vi "Run Main.vi"(8 "error in":errorcluster) -> (0 "error out":errorcluster)   [LabVIEW 2020, in "Hardware.lvlib"]
uses:
  Hardware.lvlib
  SubVIs and TypeDefs/Runtime Data.ctl
  Shared Ressources/gamepad-direction-enum.ctl
  Shared Ressources/Controller-button-pressed-enum.ctl
  <vilib>/Utility/inputDevices.llb/joystickAcquire.vi
  <userlib>/_OpenG.lib/array/array.llb/Search 1D Array (Boolean)__ogtk.vi
  <vilib>/Utility/inputDevices.llb/closeJoystick.vi
  Manager/Manager.lvlib
panel:
  out "Message Iterations":i32
  # "Message Handler: Run Main VI"
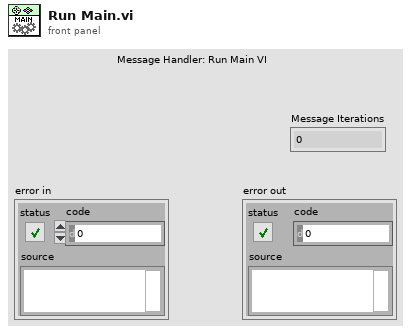
[diagram p1: front panel]
types:
  T1 = typedef "Hardware.lvlib/Runtime Data.ctl" = cluster{"ID":string, "connected?":bool, "System no.":i32, "device ID":refnum<k1>, "controller infos":cluster{"axes total":u32, "buttons total":u32, "pov total":u32, "device name":string}}
  T2 = typedef "Controller-button-pressed-enum.ctl" = enum16{"button 1", "button 2", "button 3", "button 4", "button 5", "button 6", "button 7", "button 8", "button 9", "button 10", "button 11", "button 12", "button 13", "button 14"}
  T3 = typedef "gamepad-direction-enum.ctl" = enum16{"Up Arrow", "Right Arrow", "Down Arrow", "Left Arrow"}
  T4 = cluster{"axes total":u32, "buttons total":u32, "pov total":u32, "device name":string}[]
  T5 = cluster{"axes total":u32, "buttons total":u32, "pov total":u32, "device name":string}
  T6 = cluster{"button 1":bool, "button 2":bool, "button 3":bool, "button 4":bool, "button 5":bool, "button 6":bool, "button 7":bool, "button 8":bool, "button 9":bool, "button 10":bool, "button 11":bool, "button 12":bool, "button 13":bool, "button 14":bool, "button 15":bool, "button 16":bool, "button 17":bool, "button 18":bool, "button 19":bool, "button 20":bool, "button 21":bool, "button 22":bool, "button 23":bool, "button 24":bool, "button 25":bool, "button 26":bool, "button 27":bool, "button 28":bool, "button 29":bool, "button 30":bool, "button 31":bool, "button 32":bool}
  T7 = cluster{"pov 1":i32, "pov 2":i32, "pov 3":i32, "pov 4":i32}
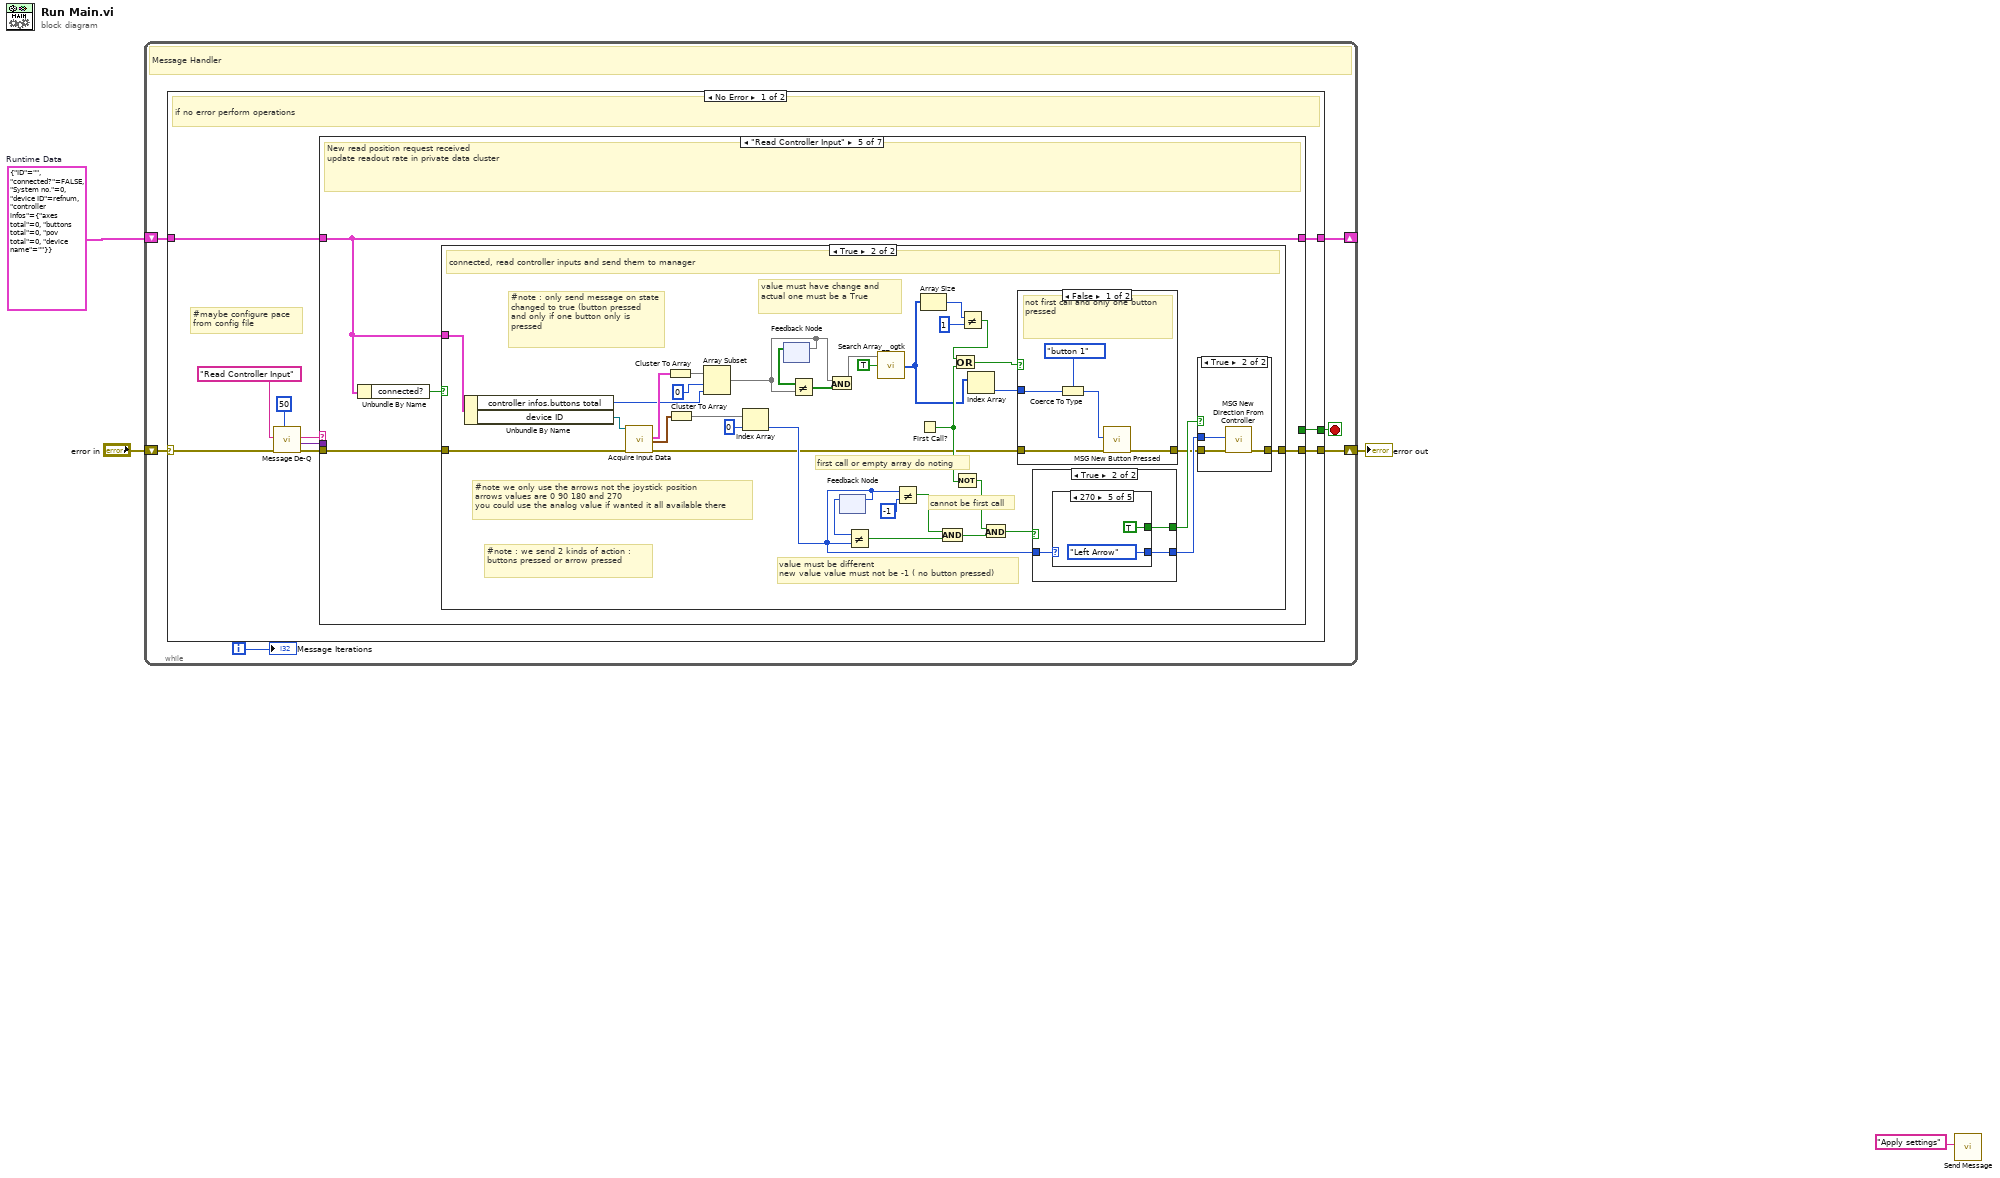
[diagram p0: block diagram]
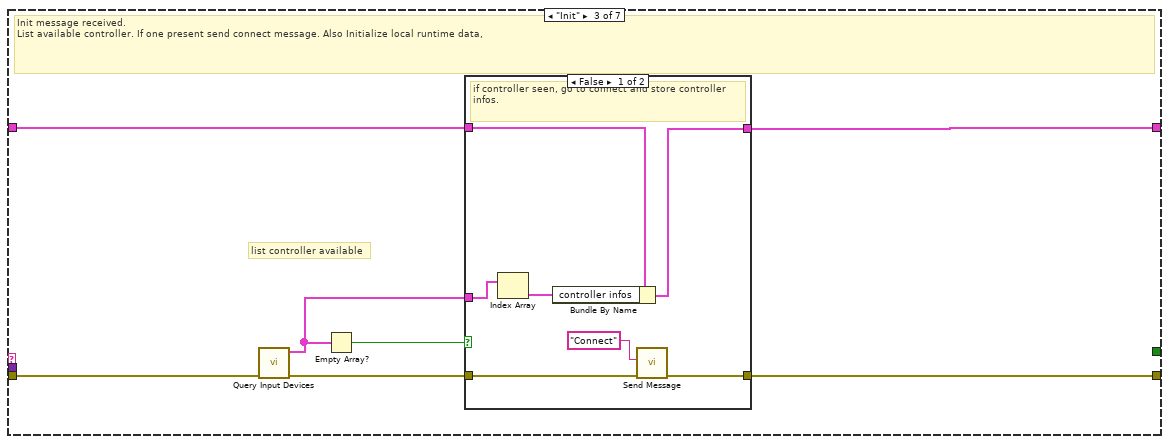
[diagram p4: hidden frame]
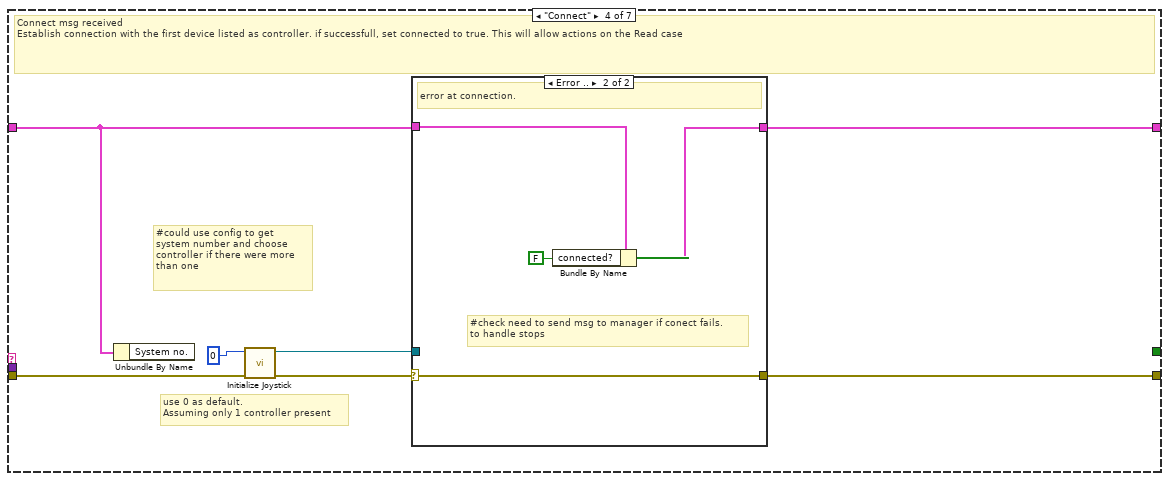
[diagram p6: hidden frame]
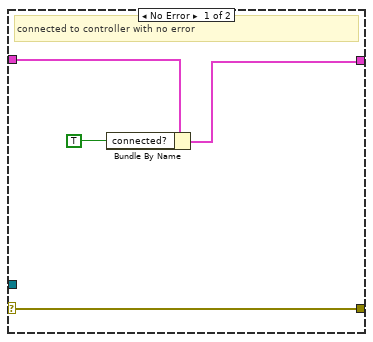
[diagram p7: hidden frame]
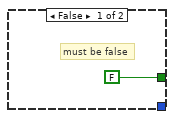
[diagram p11: hidden frame]
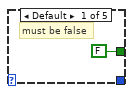
[diagram p12: hidden frame]
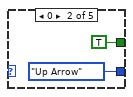
[diagram p13: hidden frame]
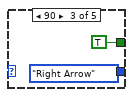
[diagram p14: hidden frame]
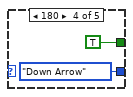
[diagram p15: hidden frame]
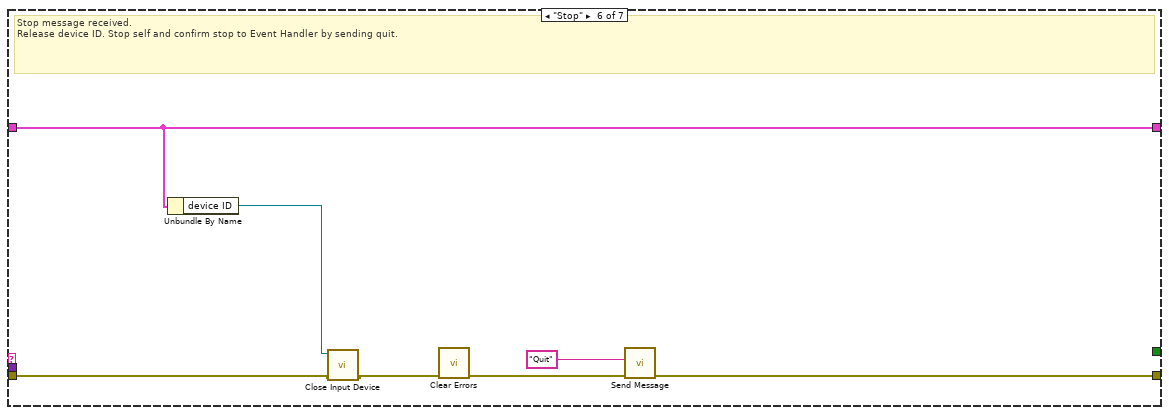
[diagram p16: hidden frame]
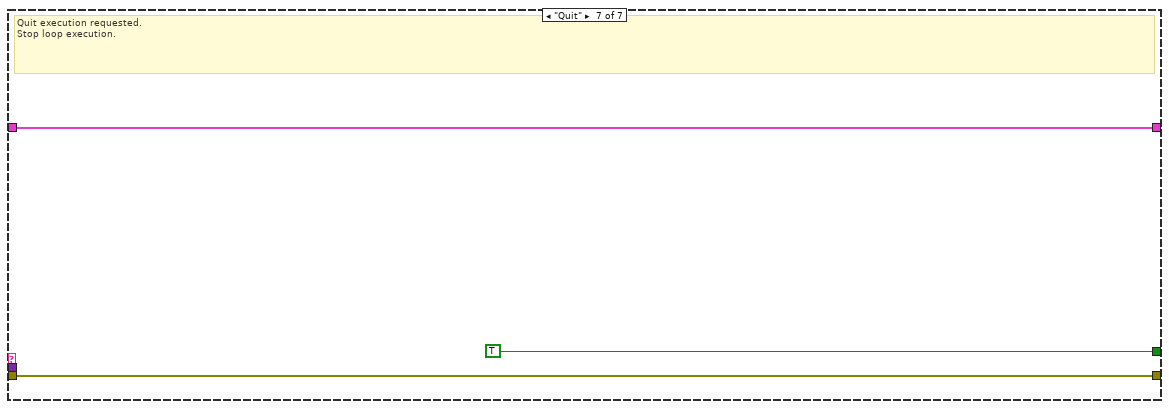
[diagram p17: hidden frame]
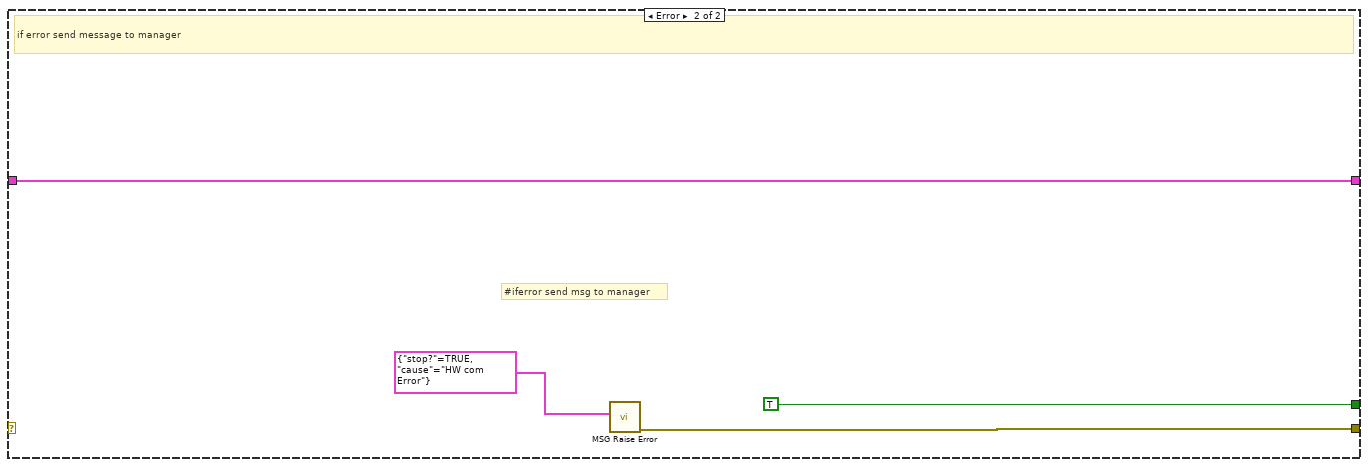
[diagram p18: hidden frame]
diagram:
  w1 = T1 {"ID"="", "connected?"=FALSE, "System no."=0, "device ID"=refnum, "controller infos"={"axes total"=0, "buttons total"=0, "pov total"=0, "device name"=""}}  # Runtime Data
  n1 = while {
    shift-right: [w8] -> w3
    shift-left: "error in" -> [w5]
    shift-right: [w6] -> _
    shift-left: w1 -> [w9]
    i -> [w10]
    stop <- w7 stop-if-true
    # "Message Handler"
    n2 = case shown="No Error" w5 {
      selector: w5 -> [w12 _]
      tunnel: w9 -> [w13 w131]
      tunnel: [w17 w129] -> w8
      tunnel: [w16 TRUE] -> w7
      tunnel: [w15 w131] -> w6
      frame No Error {
        # "#maybe configure pace\nfrom config file"
        # "if no error perform operations"
        n3 = call "Message De-Q.vi"("timeout [ms]"=50, "error in"=w12, "timeout cmd"="Read Controller Input") -> ("error out"=w18:errorcluster, "Payload"=w19:variant, "Command"=w20:string)  [unwired: 5 in, 1 out]
        n4 = case shown="\"Read Controller Input\"" w20 {
          tunnel: [w22 w23 w31 w47 w58 w124 w128] -> w17
          tunnel: w18 -> [w22 w23 w30 w44 w59 w120 w128]
          tunnel: [_ _ _ _ _ _ TRUE] -> w16
          tunnel: [w21 w24 w25 w46 w56 w123 w126] -> w15
          tunnel: w13 -> [w21 w24 w26 w41 w56 w123 w126]
          tunnel: w19 -> [_ _ _ _ _ _ _]
          frame Default {
            # "Message not recognized.\nDevelopment time error. Message not recognized. Maybe a typo? Pop up a blocking dialog for the developer to be informed about the situation."
          }
          frame "Message Timeout" {
            # "Message queue timeout.\nThis case is executed regularly when the messaging queue is empty.\nThink: IDLE."
          }
          frame "Init" {
            # "list controller available"
            # "Init message received.\nList available controller. If one present send connect message. Also Initialize local runtime data,"
            n5 = call <vilib>:"Query Input Devices.vi"("error in (no error)"=w30) -> ("error out"=w29:errorcluster, "joystick info"=w27:T4)  [unwired: 7 in, 2 out]
            n6 = Empty Array?(array=w27) -> (empty?=w28:bool)
            n7 = case shown="False" w28 {
              tunnel: [w37 w40] -> w31
              tunnel: w29 -> [w36 w40]
              tunnel: w27 -> [w35 _]
              tunnel: w26 -> [w33 w39]
              tunnel: [w32 w39] -> w25
              frame False {
                # "if controller seen, go to connect and store controller infos."
                n8 = Index Array(array=w35) -> (element=w34:T5)  [unwired: 1 in]
                n9 = Bundle By Name(cluster=w33, "controller infos"=w34) -> (w32:T1)
                n10 = call "Send Message.vi"("error in"=w36, "Command"="Connect") -> ("error out"=w37:errorcluster)  [unwired: 9 in]
              }
              frame True {
                # "#report no Controller connected"
              }
            }
          }
          frame "Connect" {
            # "use 0 as default.\nAssuming only 1 controller present"
            # "#could use config to get system number and choose controller if there were more than one"
            # "Connect msg received\nEstablish connection with the first device listed as controller. if successfull, set connected to true. This will allow actions on the Read case"
            n11 = Unbundle By Name(w41) -> ()  [unwired: 1 out]
            n12 = call <vilib>:"Initialize Joystick.vi"("error in (no error)"=w44, "device index"=0) -> ("error out"=w43:errorcluster, "device ID"=w42:refnum<k1>)  [unwired: 8 in]
            n13 = case shown="Error .." w43 {
              selector: w43 -> [w48 w55]
              tunnel: [w48 w55] -> w47
              tunnel: w41 -> [w51 w54]
              tunnel: [w50 w52] -> w46
              tunnel: w42 -> [_ _]
              frame No Error {
                # "connected to controller with no error"
                n14 = Bundle By Name(cluster=w51, "connected?"=TRUE) -> (w50:T1)
              }
              frame Error {
                # "#check need to send msg to manager if conect fails.\nto handle stops"
                # "error at connection."
                n15 = Bundle By Name(cluster=w54, "connected?"=FALSE) -> (w52:T1)
              }
            }
          }
          frame "Read Controller Input" {
            # "New read position request received\nupdate readout rate in private data cluster"
            n16 = Unbundle By Name(w56) -> ("connected?"=w57:bool)
            n17 = case shown="True" w57 {
              tunnel: w59 -> [w60 w95]
              tunnel: [w60 w72] -> w58
              tunnel: w56 -> [_ w94]
              frame False {
                # "not connected yet, do nothing"
              }
              frame True {
                # "#note : we send 2 kinds of action : buttons pressed or arrow pressed"
                # "#note we only use the arrows not the joystick position\narrows values are 0 90 180 and 270\nyou could use the analog value if wanted it all available there"
                # "#note : only send message on state changed to true (button pressed and only if one button only is pressed"
                # "cannot be first call"
                # "value must be different\nnew value value must not be -1 ( no button pressed)"
                # "first call or empty array do noting"
                # "value must have change and actual one must be a True"
                # "connected, read controller inputs and send them to manager"
                n18 = Unbundle By Name(w94) -> ("controller infos.buttons total"=w89:u32, "device ID"=w93:refnum<k1>)
                n19 = call-poly <vilib>:"Acquire Input Data.vi"("device ID"=w93, "error in (no error)"=w95) -> ("button info"=w92:T6, "direction info"=w88:T7, "error out"=w64:errorcluster)  [unwired: 13 in, 2 out]
                n20 = Cluster To Array(cluster=w92) -> (array=w91:bool[])
                n21 = Cluster To Array(cluster=w88) -> (array=w82:i32[])
                n22 = Array Subset(array=w91, index=0, length=w89) -> (w85:bool[])
                n23 = Index Array(array=w82, index=0) -> (element=w74:i32)
                n24 = feedback-in #1(w85) -> ()
                n25 = feedback #1() -> (w87:bool[])  [unwired: 1 in]
                n26 = Not Equal?(x=w87, y=w85) -> (x != y?=w86:bool[])
                n27 = And(x=w85, y=w86) -> (x .and. y?=w84:bool[])
                n28 = feedback #2() -> (w81:i32)  [unwired: 1 in]
                n29 = feedback-in #2(w74) -> ()
                n30 = Not Equal?(x=w81, y=w74) -> (x != y?=w80:bool)
                n31 = call-poly <userlib>:"Search Array__ogtk.vi"("Array"=w84, "Element Data"=TRUE) -> ("Indices of Elements"=w66:i32[])  [unwired: 7 in]
                n32 = Not Equal?(x=w74, y=-1) -> (x != y?=w79:bool)
                n33 = First Call?() -> (First Call?: T/F=w69:bool)
                n34 = Array Size(array=w66) -> (size(s)=w70:i32)
                n35 = And(x=w79, y=w80) -> (x .and. y?=w76:bool)
                n36 = Not(x=w69) -> (.not. x?=w77:bool)
                n37 = Not Equal?(x=w70, y=1) -> (x != y?=w68:bool)
                n38 = Or(x=w68, y=w69) -> (x .or. y?=w71:bool)
                n39 = Index Array(array=w66) -> (element=w65:i32)  [unwired: 1 in]
                n40 = And(x=w77, y=w76) -> (x .and. y?=w75:bool)
                n41 = case shown="False" w71 {
                  tunnel: w65 -> [w99 _]
                  tunnel: w64 -> [w97 w101]
                  tunnel: [w96 w101] -> w62
                  frame False {
                    # "not first call and only one button pressed"
                    n42 = Coerce To Type(0:w99, 1:Controller-button-pressed-enum."button 1") -> (2:w98:T2)
                    n43 = call "MSG New Button Pressed.vi"("error in"=w97, "data"=w98) -> ("error out"=w96:errorcluster)  [unwired: 9 in]
                  }
                  frame True {
                    # "first call, no button touched, or more than one, do nothing"
                  }
                }
                n44 = case shown="True" w75 {
                  tunnel: w74 -> [_ w109]
                  tunnel: [FALSE w108] -> w73
                  tunnel: [_ w107] -> w63
                  frame False {
                    # "must be false"
                  }
                  frame True {
                    n45 = case shown="270" w109 {
                      tunnel: [FALSE TRUE TRUE TRUE TRUE] -> w108
                      tunnel: [_ gamepad-direction-enum."Up Arrow" gamepad-direction-enum."Right Arrow" gamepad-direction-enum."Down Arrow" gamepad-direction-enum."Left Arrow"] -> w107
                      frame Default {
                        # "must be false"
                      }
                      frame 0 {
                      }
                      frame 90 {
                      }
                      frame 180 {
                      }
                      frame 270 {
                      }
                    }
                  }
                }
                n46 = case shown="True" w73 {
                  tunnel: [w102 w105] -> w72
                  tunnel: w63 -> [_ w104]
                  tunnel: w62 -> [w102 w103]
                  frame False {
                  }
                  frame True {
                    n47 = call "MSG New Direction From Controller.vi"("error in"=w103, "data"=w104) -> ("error out"=w105:errorcluster)  [unwired: 9 in]
                  }
                }
              }
            }
          }
          frame "Stop" {
            # "Stop message received.\nRelease device ID. Stop self and confirm stop to Event Handler by sending quit."
            n48 = Unbundle By Name(w123) -> ("device ID"=w121:refnum<k1>)
            n49 = call-poly <vilib>:"Close Input Device.vi"("error in (no error)"=w120, "device ID"=w121) -> ("error out"=w119:errorcluster)  [unwired: 8 in]
            n50 = call <vilib>:"Clear Errors.vi"("error in (no error)"=w119) -> ("error out"=w122:errorcluster)  [unwired: 5 in, 1 out]
            n51 = call "Send Message.vi"("error in"=w122, "Command"="Quit") -> ("error out"=w124:errorcluster)  [unwired: 9 in]
          }
          frame "Quit" {
            # "Quit execution requested.\nStop loop execution."
          }
        }
      }
      frame Error {
        # "#iferror send msg to manager"
        # "if error send message to manager"
        n52 = call "MSG Raise Error.vi"("raised error"=cluster{"stop?":bool, "cause":string} {"stop?"=TRUE, "cause"="HW com Error"}) -> ("error out"=w129:errorcluster)  [unwired: 10 in]
      }
    }
    "Message Iterations" <- w10
  }
  "error out" <- w3
  n53 = call "Send Message.vi"("Command"="Apply settings") -> ()  [unwired: 10 in, 1 out]
